vi "nanocal -- nuclear schottky fit V3.vi"() -> ()   [LabVIEW 2020] (continued)
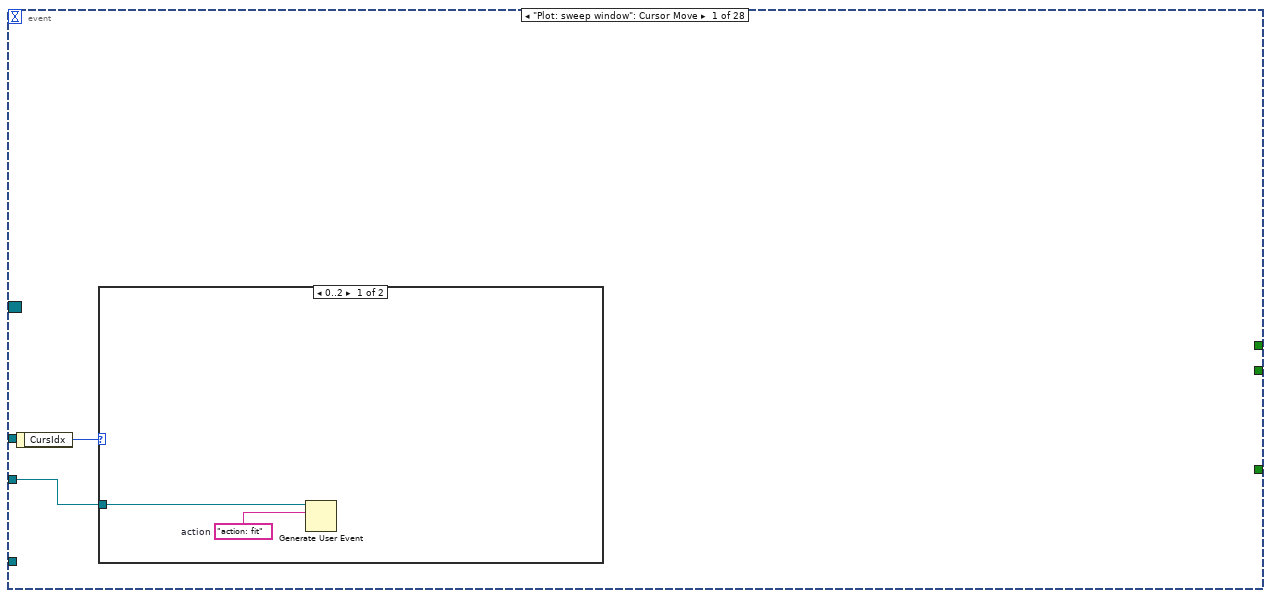
[diagram p2: hidden frame]
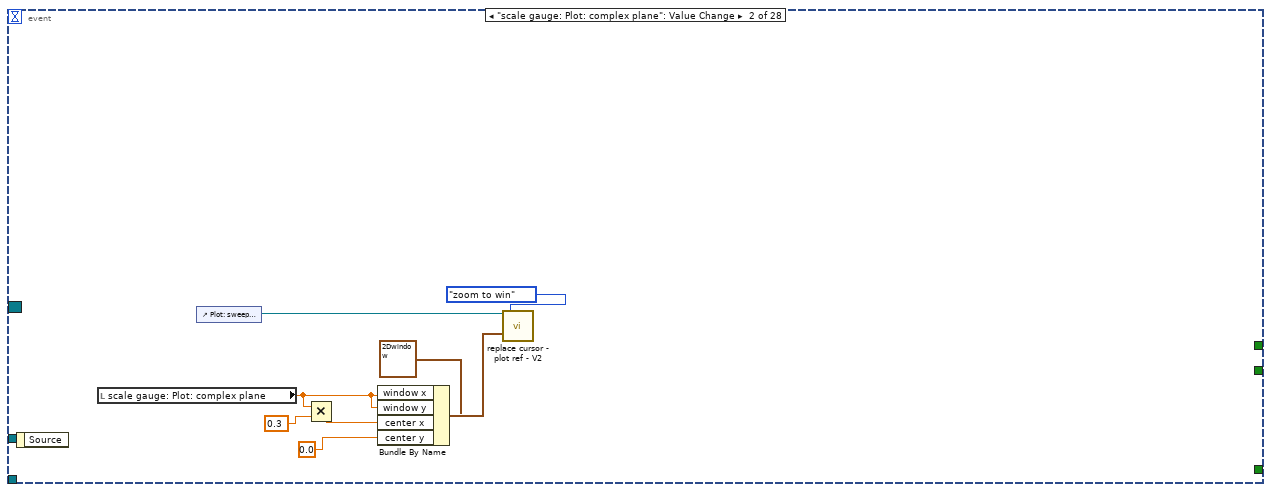
[diagram p4: hidden frame]
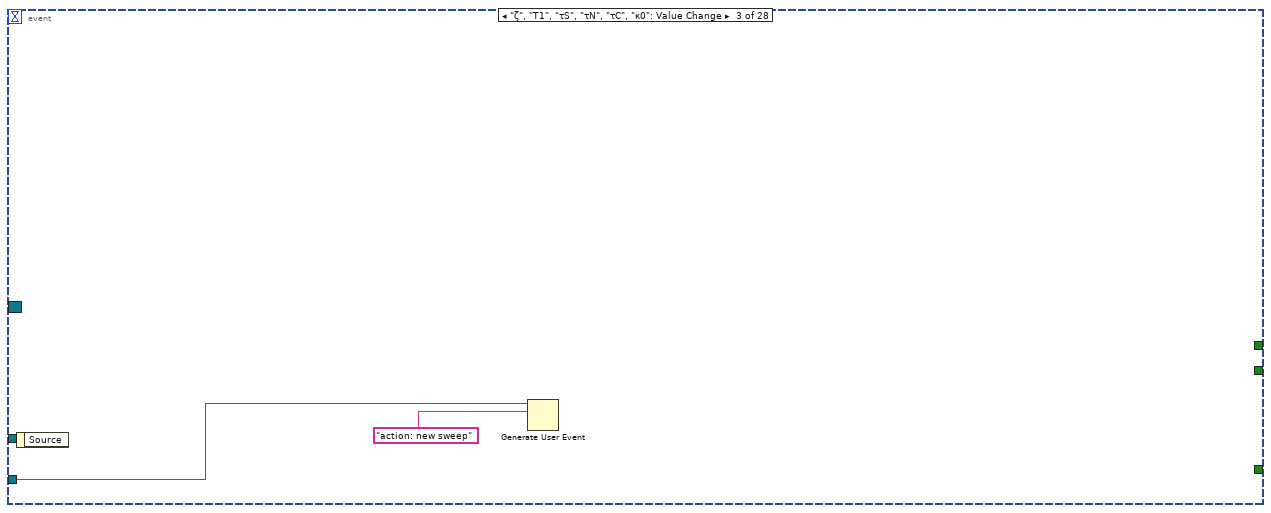
[diagram p5: hidden frame]
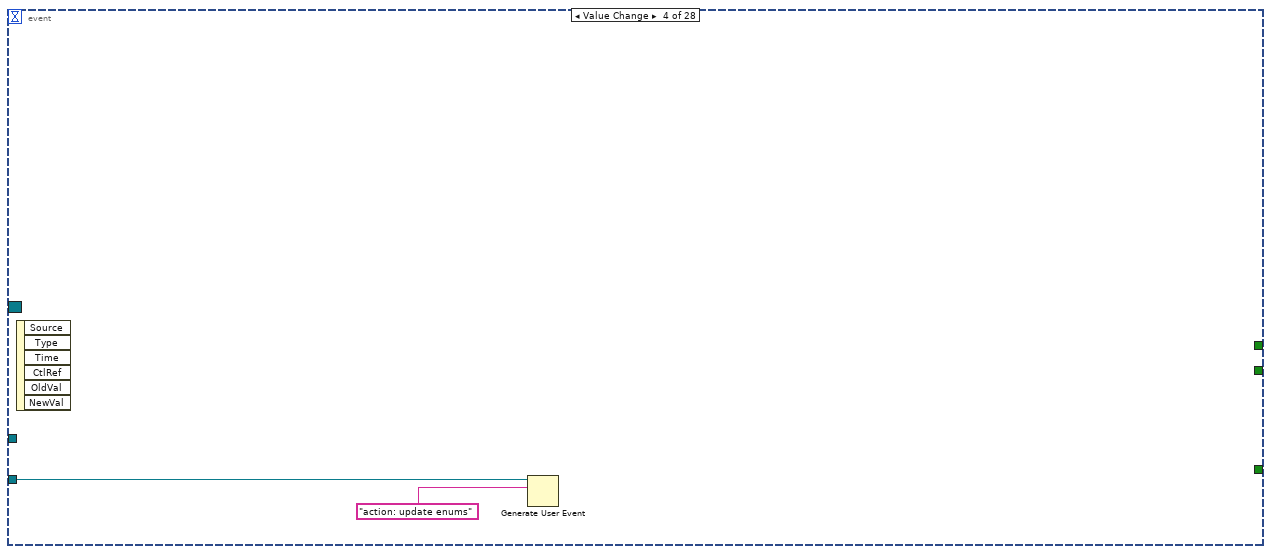
[diagram p6: hidden frame]
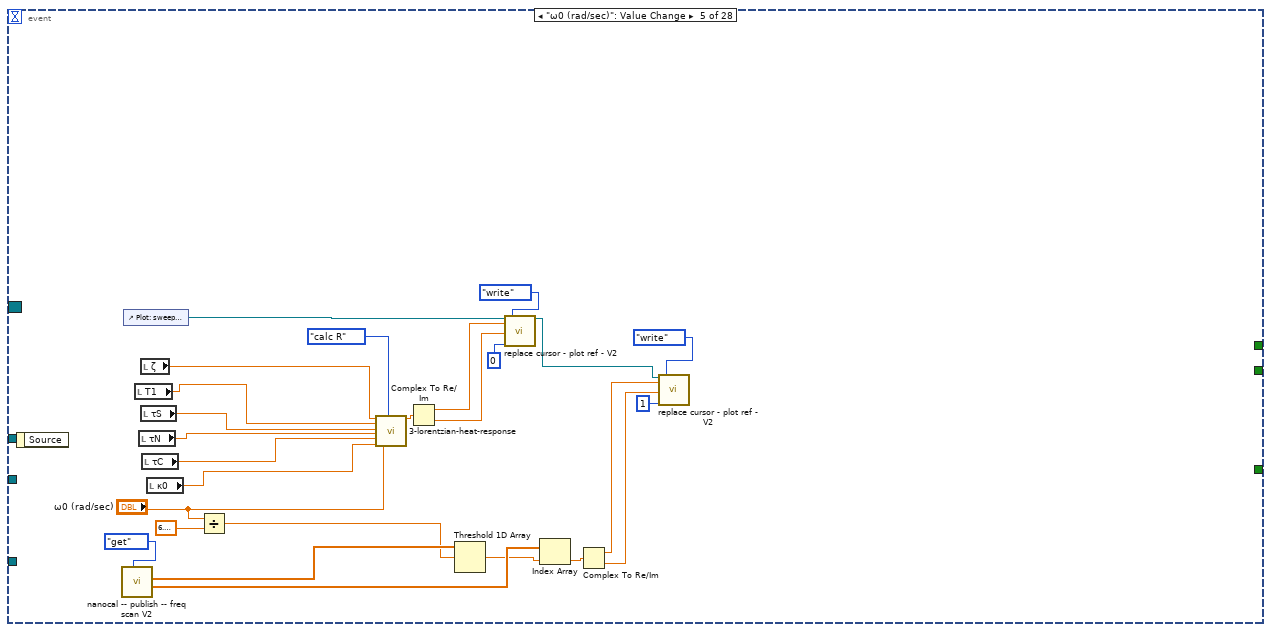
[diagram p7: hidden frame]
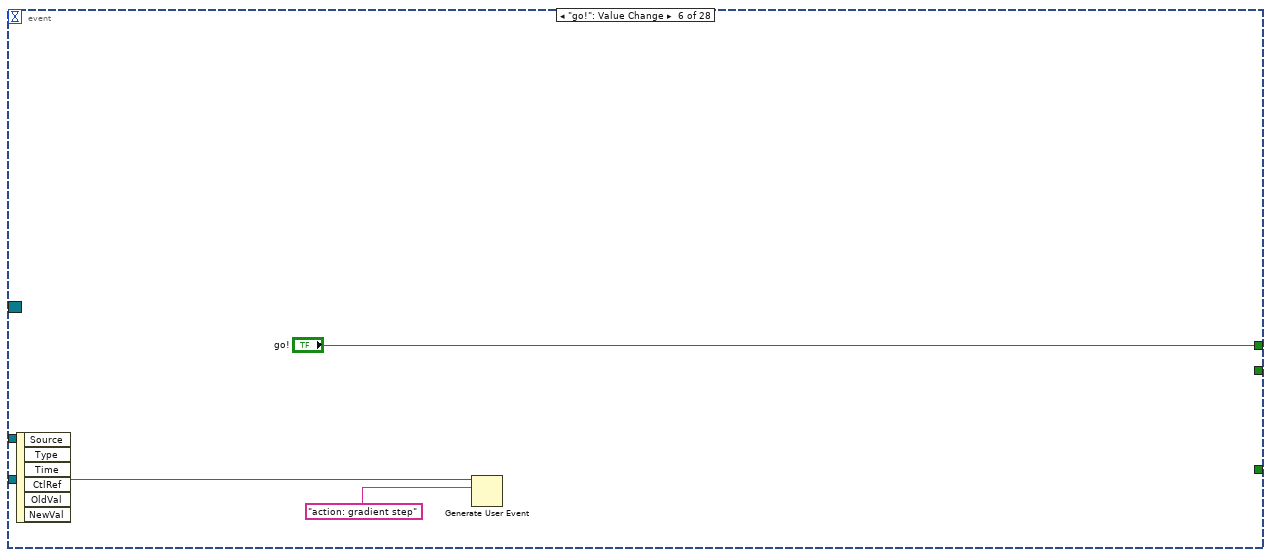
[diagram p8: hidden frame]
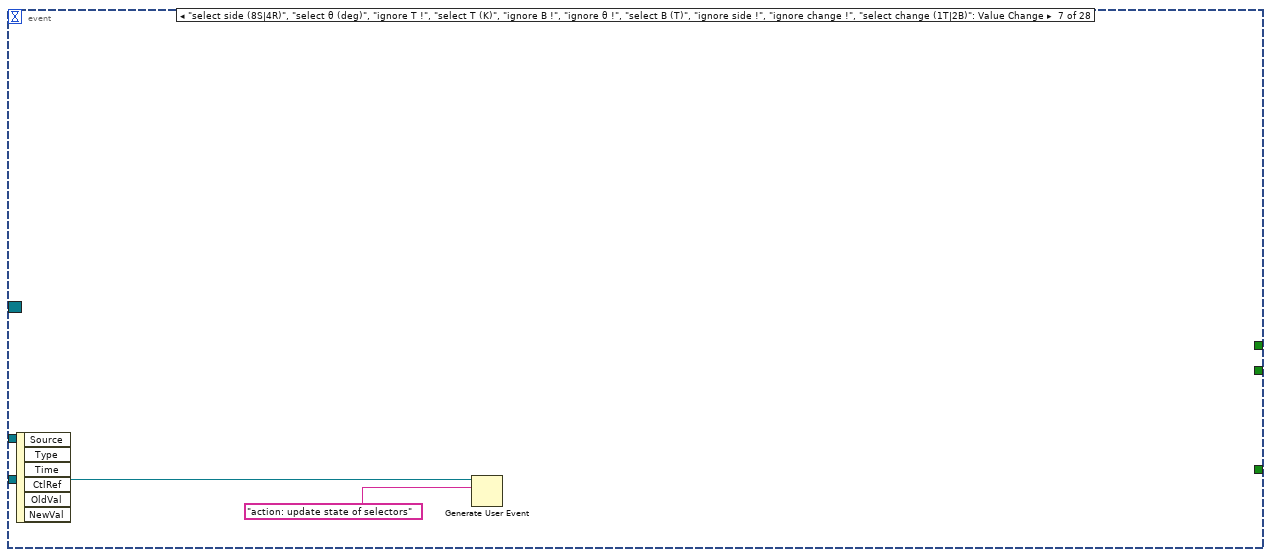
[diagram p9: hidden frame]
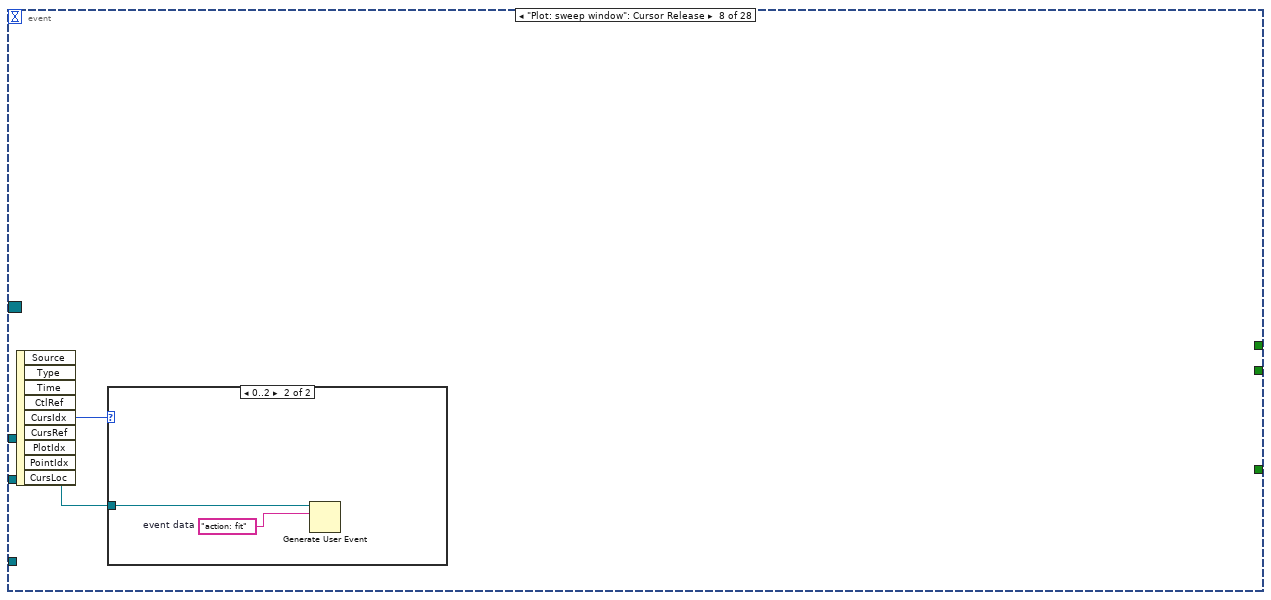
[diagram p10: hidden frame]
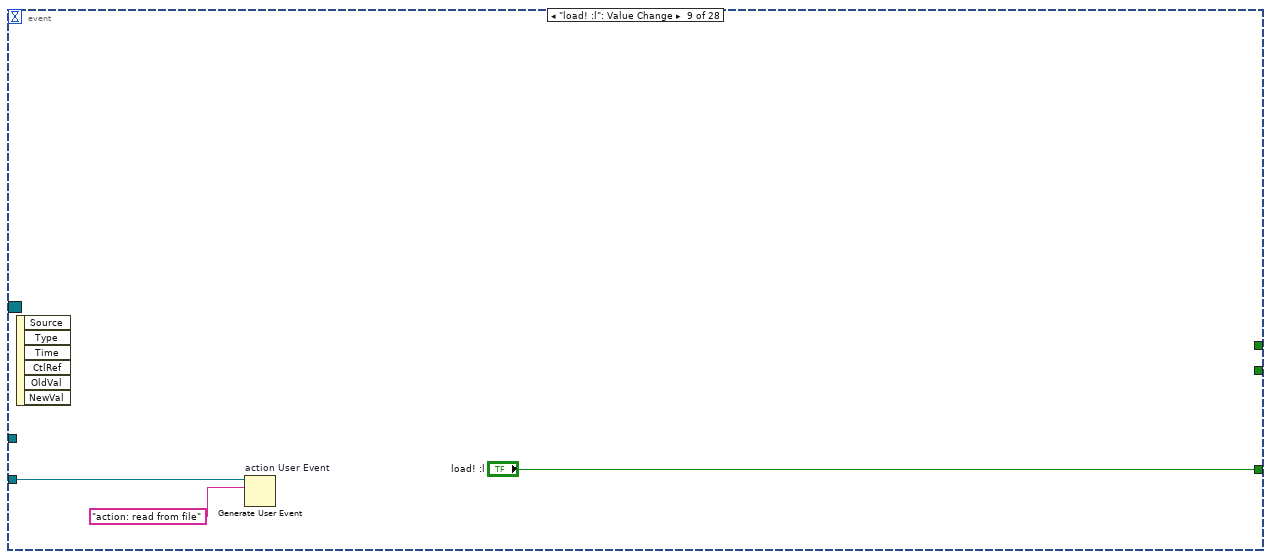
[diagram p12: hidden frame]
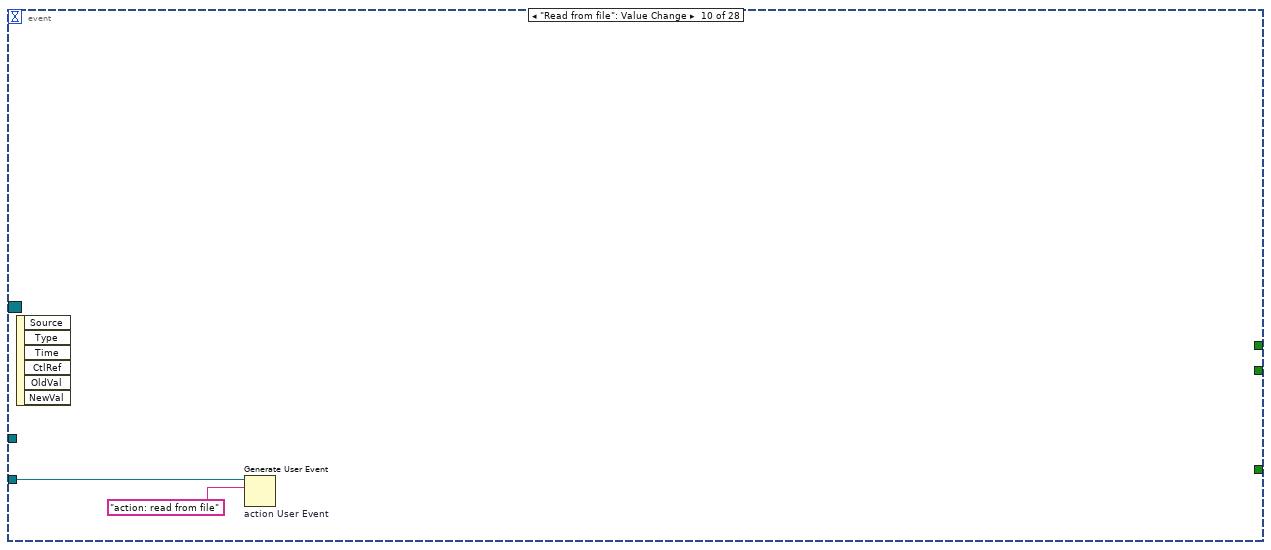
[diagram p13: hidden frame]
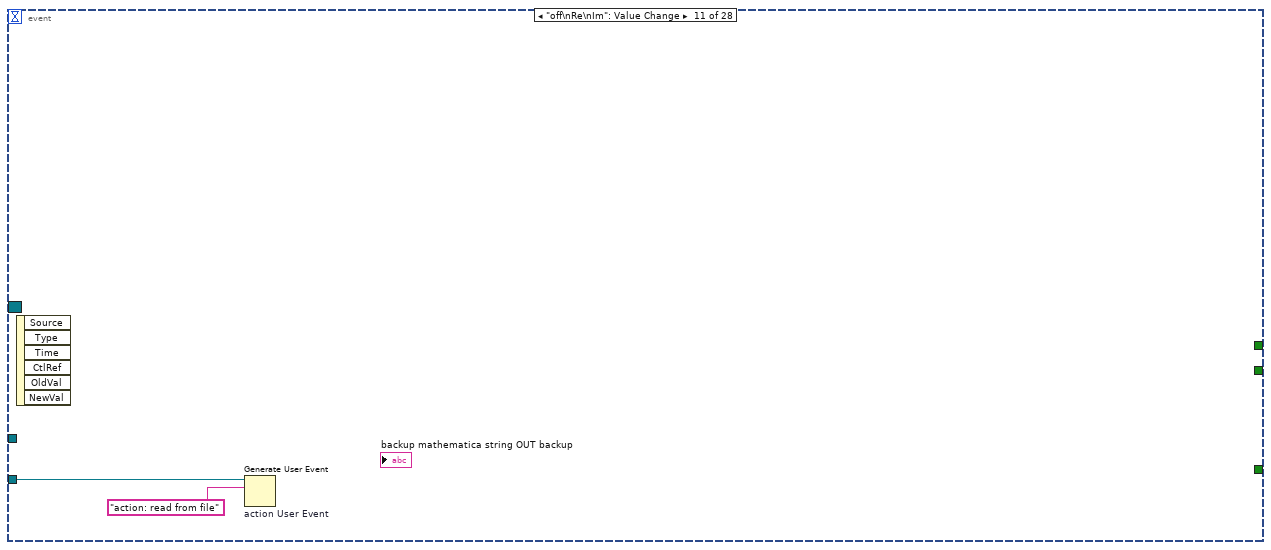
[diagram p14: hidden frame]
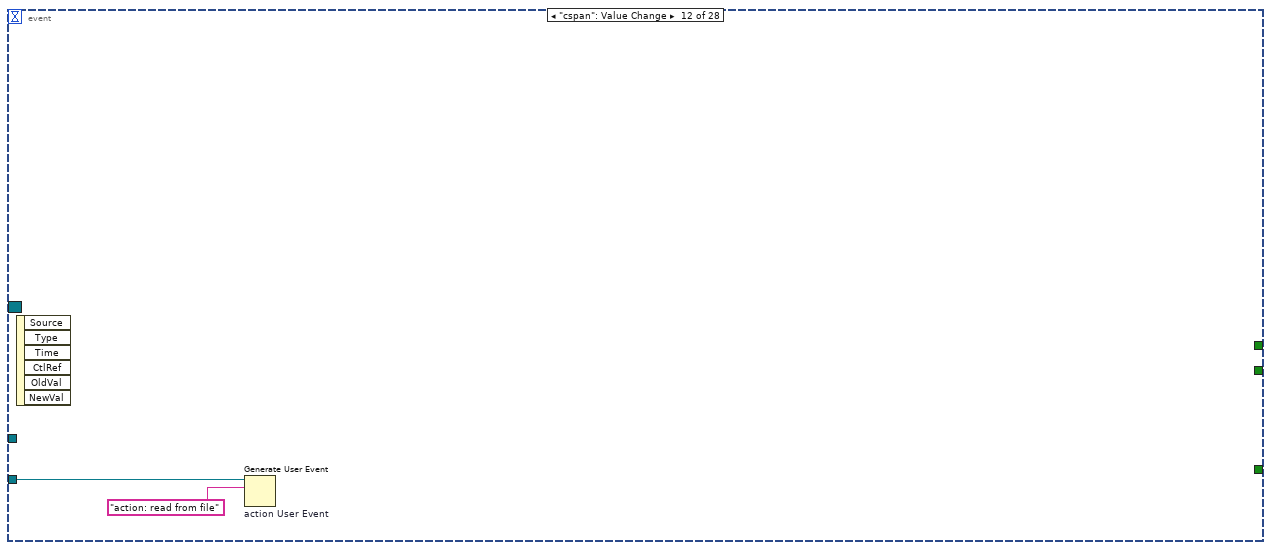
[diagram p15: hidden frame]
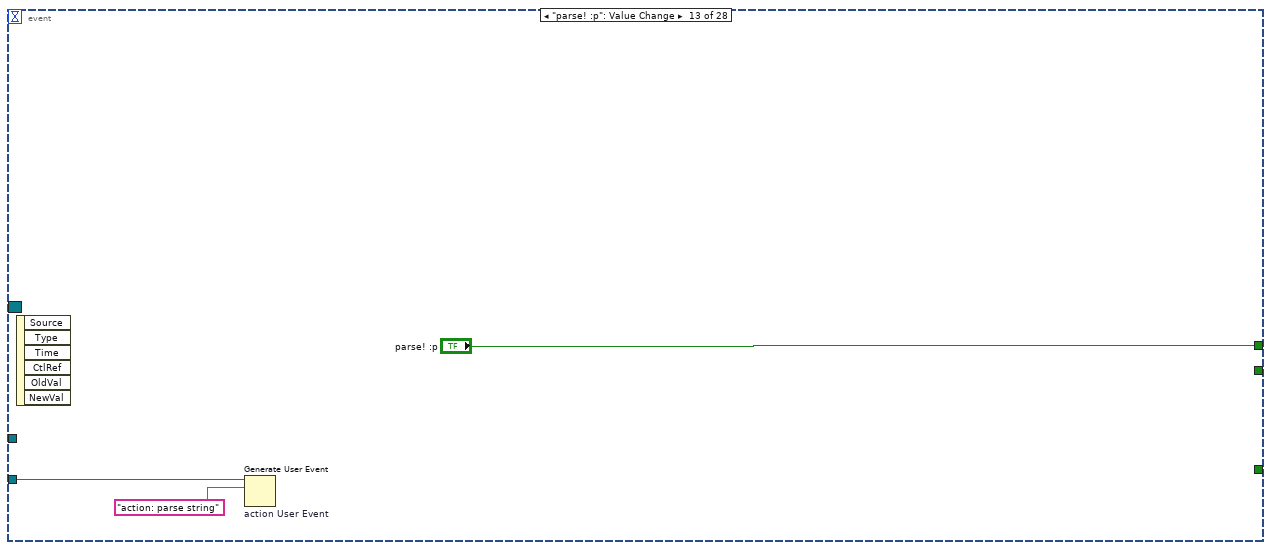
[diagram p16: hidden frame]
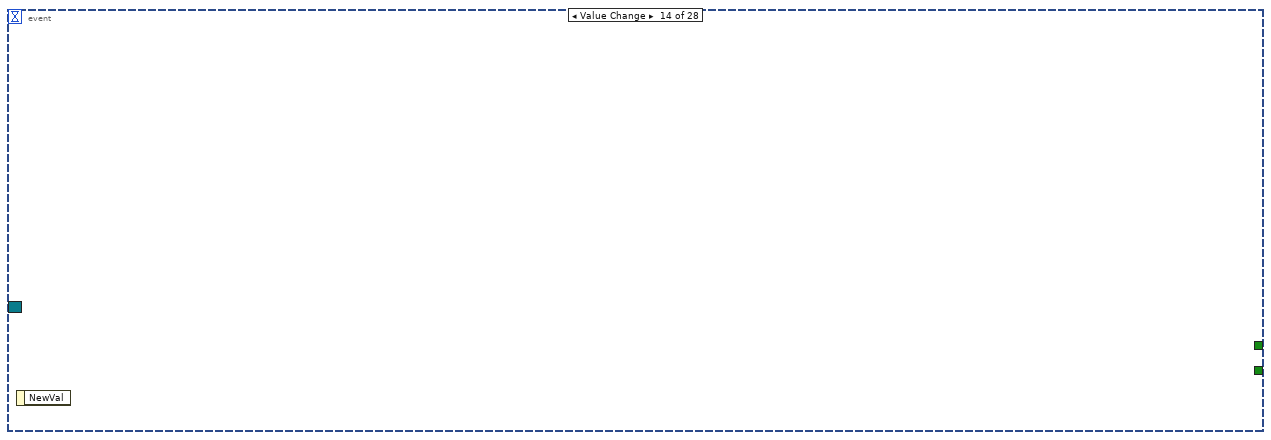
[diagram p17: hidden frame]
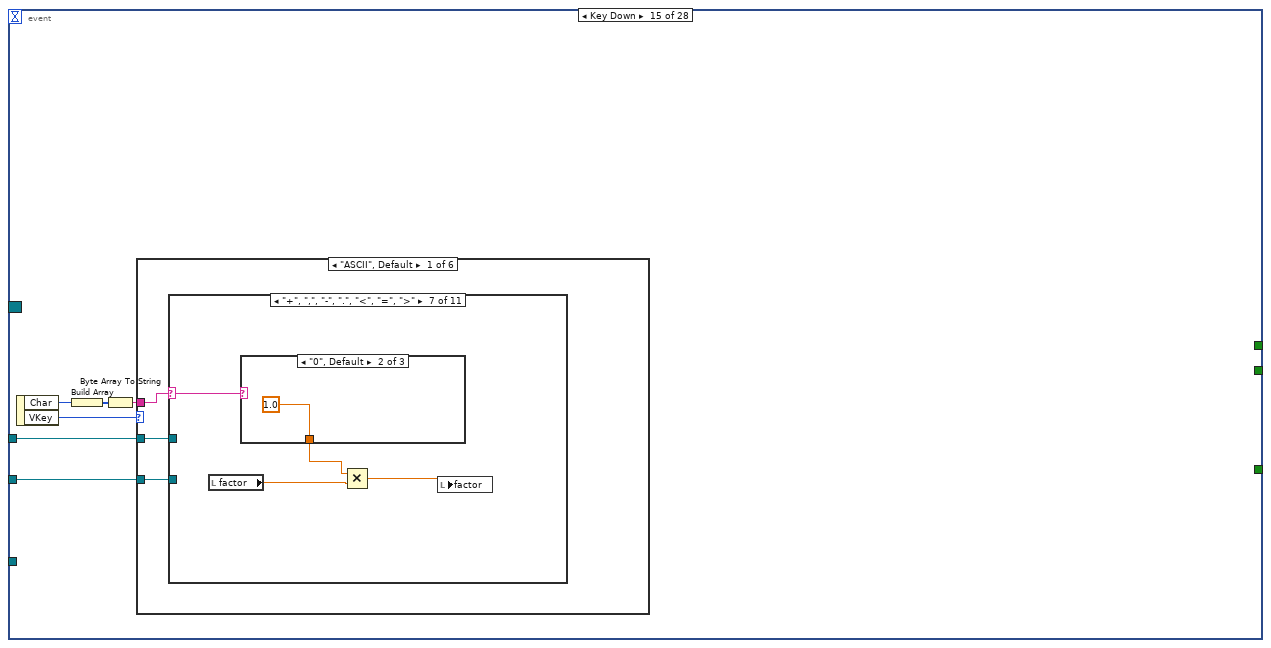
[diagram p18: hidden frame]
      event "ω0 (rad/sec)": Value Change {
        n583 = event-data() -> ()  [unwired: 1 in, 1 out]
        n584 = call "nanocal -- publish -- freq scan V2.vi"("publisher action"=publisher_action."get") -> ("z out (V)"=w1143:cdb[], "ω out (Hz)"=w1138:dbl[])  [unwired: 8 in, 1 out]
        n585 = control-ref of="Plot: sweep window"() -> (w1125:refnum<vi>)
        n586 = local read "T1"() -> (w1127:dbl)
        n587 = local read "τN"() -> (w1129:dbl)
        n588 = local read "ζ"() -> (w1126:dbl)
        n589 = local read "τS"() -> (w1128:dbl)
        n590 = local read "τC"() -> (w1130:dbl)
        n591 = local read "κ0"() -> (w1131:dbl)
        n592 = Divide(x="ω0 (rad/sec)", y=6.283185307179586) -> (x/y=w1136:dbl)
        n593 = call "3-lorentzian-heat-response.vi"("zeta"=w1126, "T1"=w1127, "tauS"=w1128, "tauN"=w1129, "tauC"=w1130, "kappa0"=w1131, "omega (rad/sec)"="ω0 (rad/sec)", "action"=3-lorentzian-heat-response_action."calc R") -> ("Romega"=w1134:cdb)  [unwired: 7 in, 4 out]
        n594 = Complex To Re/Im(x + iy=w1134) -> (x=w1132:dbl, y=w1133:dbl)
        n595 = Threshold 1D Array(2:w1136, 3:w1138) -> (0:w1137:dbl)  [unwired: 1 in]
        n596 = call "replace cursor - plot ref - V2.vi"("Plot ref in"=w1125, "new X"=w1132, "new  Y"=w1133, "cursor index"=0, "cursor action"=cursor_action."write") -> ("Plot ref out"=w1139:refnum<vi>)  [unwired: 11 in, 3 out]
        n597 = Index Array(array=w1143, index=w1137) -> (element=w1140:cdb)
        n598 = Complex To Re/Im(x + iy=w1140) -> (x=w1141:dbl, y=w1142:dbl)
        n599 = call "replace cursor - plot ref - V2.vi"("Plot ref in"=w1139, "new X"=w1141, "new  Y"=w1142, "cursor index"=1, "cursor action"=cursor_action."write") -> ()  [unwired: 11 in, 4 out]
      }
      event "go!": Value Change {
        n600 = event-data() -> ()  [unwired: 1 in, 6 out]
        n601 = Generate User Event(user event=w1145, event data cluster="action: gradient step" ("event data")) -> ()  [unwired: 2 in, 2 out]
      }
      event "select side (8S|4R)", "select θ (deg)", "ignore T !", "select T (K)", "ignore B !", "ignore θ !", "select B (T)", "ignore side !", "ignore change !", "select change (1T|2B)": Value Change {
        n602 = event-data() -> ()  [unwired: 1 in, 6 out]
        n603 = Generate User Event(user event=w1147, event data cluster="action: update state of selectors" ("event data")) -> ()  [unwired: 2 in, 2 out]
      }
      event "Plot: sweep window": Cursor Release {
        n604 = event-data() -> ("CursIdx"=w1149:i32)  [unwired: 1 in, 8 out]
        n605 = case shown="0..2" w1149 {
          tunnel: w1150 -> [_ w1151]
          frame 3, Default {
          }
          frame 0..2 {
            w1152 = "action: fit"  # event data
            n606 = Generate User Event(user event=w1151, event data cluster=w1152) -> ()  [unwired: 2 in, 2 out]
          }
        }
      }
      event "load! :l": Value Change {
        n607 = event-data() -> ()  [unwired: 1 in, 6 out]
        n608 = Generate User Event "action User Event"(user event=w1155, event data cluster="action: read from file" ("event data")) -> ()  [unwired: 2 in, 2 out]
      }
      event "Read from file": Value Change {
        n609 = event-data() -> ()  [unwired: 1 in, 6 out]
        n610 = Generate User Event "action User Event"(user event=w1156, event data cluster="action: read from file" ("event data")) -> ()  [unwired: 2 in, 2 out]
      }
      event "off\nRe\nIm": Value Change {
        n611 = event-data() -> ()  [unwired: 1 in, 6 out]
        n612 = Generate User Event "action User Event"(user event=w1158, event data cluster="action: read from file" ("event data")) -> ()  [unwired: 2 in, 2 out]
      }
      event "cspan": Value Change {
        n613 = event-data() -> ()  [unwired: 1 in, 6 out]
        n614 = Generate User Event "action User Event"(user event=w1160, event data cluster="action: read from file" ("event data")) -> ()  [unwired: 2 in, 2 out]
      }
      event "parse! :p": Value Change {
        n615 = event-data() -> ()  [unwired: 1 in, 6 out]
        n616 = Generate User Event "action User Event"(user event=w1163, event data cluster="action: parse string" ("event data")) -> ()  [unwired: 2 in, 2 out]
      }
      event Value Change {
        n617 = event-data() -> ()  [unwired: 1 in, 1 out]
      }
      event Key Down {
        n618 = event-data() -> ("Char"=w1167:i16, "VKey"=w1170:T28)  [unwired: 1 in]
        n619 = Build Array(w1167) -> (w1168:i16[])
        n620 = Byte Array To String(unsigned byte array=w1168) -> (string=w1166:string)
        n621 = case shown="\"ASCII\", Default" w1170 {
          selector: w1170 -> [_ _ _ _ _ w1202]
          tunnel: w1169 -> [w1173 _ _ w1198 _ _]
          tunnel: w1166 -> [w1172 _ _ _ _ _]
          tunnel: w1165 -> [w1171 _ _ _ _ w1201]
          frame "ASCII", Default {
            n622 = case shown="\"+\", \",\", \"-\", \".\", \"<\", \"=\", \">\"" w1172 {
              selector: w1172 -> [_ _ _ _ _ _ w1185 _ _ _ _]
              tunnel: w1173 -> [_ _ w1174 w1176 w1179 _ _ _ w1192 w1194 w1196]
              tunnel: w1171 -> [_ _ _ _ _ w1183 _ _ _ _ _]
              frame "0", Default {
              }
              frame "a" {
              }
              frame "s" {
                n623 = Generate User Event(user event=w1174, event data cluster="action: save freq scan" ("event data")) -> ()  [unwired: 2 in, 2 out]
              }
              frame "l" {
                n624 = Generate User Event(user event=w1176, event data cluster="action: read from file" ("event data")) -> ()  [unwired: 2 in, 2 out]
              }
              frame " " {
                n625 = Generate User Event(user event=w1179, event data cluster="action: gradient step" ("event data")) -> ()  [unwired: 2 in, 2 out]
              }
              frame "?" {
                # "?"
                n626 = call "replace cursor - plot ref - V2.vi"("Plot ref in"=w1183, "cursor action"=cursor_action."zoom to win") -> ("Plot ref out"=w1182:refnum<vi>)  [unwired: 14 in, 3 out]
                n627 = call "replace cursor - plot ref - V2.vi"("Plot ref in"=w1182, "cursor action"=cursor_action."smart zoom out&aspect") -> ()  [unwired: 14 in, 4 out]
              }
              frame "+", ",", "-", ".", "<", "=", ">" {
                n628 = local read "factor"() -> (w1187:dbl)
                n629 = case shown="\"0\", Default" w1185 {
                  tunnel: [0.7 1.0 1.5] -> w1184
                  frame ",", "-", "<" {
                  }
                  frame "0", Default {
                  }
                  frame "+", ".", "=", ">" {
                  }
                }
                n630 = Multiply(x=w1184, y=w1187) -> (x*y=w1186:dbl)
                n631 = local write "factor"(w1186) -> ()
              }
              frame "b" {
                n632 = local read "String"() -> (w1191:string)
                n633 = local write "backup string :b"(w1191) -> ()
              }
              frame "u" {
                n634 = Generate User Event(user event=w1192, event data cluster="ignoreaction: uco" ("event data")) -> ()  [unwired: 2 in, 2 out]
              }
              frame "p" {
                n635 = Generate User Event "action User Event"(user event=w1194, event data cluster="action: parse string" ("event data")) -> ()  [unwired: 2 in, 2 out]
              }
              frame "m" {
                n636 = Generate User Event "action User Event"(user event=w1196, event data cluster="action: copy from math" ("event data")) -> ()  [unwired: 2 in, 2 out]
              }
            }
          }
          frame "Escape" {
          }
          frame "PageUp" {
          }
          frame "Enter" {
            n637 = Generate User Event "action User Event"(user event=w1198, event data cluster="action: replot colors" ("event data")) -> ()  [unwired: 2 in, 2 out]
            n638 = Generate User Event "action User Event"(user event=w1198, event data cluster="action: new sweep" ("event data")) -> ()  [unwired: 2 in, 2 out]
          }
          frame "PageDown" {
          }
          frame "Up".."Right" {
            n639 = case shown="\"Down\"" w1202 {
              tunnel: [cursor_action."zoom in 20%" ("cursor action") cursor_action."zoom out 20%" ("cursor action") cursor_action."zoom out 20%" ("cursor action") cursor_action."zoom in 20%" ("cursor action")] -> w1203
              frame "Up", Default {
              }
              frame "Down" {
              }
              frame "Left" {
              }
              frame "Right" {
              }
            }
            n640 = call "replace cursor - plot ref - V2.vi"("Plot ref in"=w1201, "cursor action"=w1203) -> ()  [unwired: 14 in, 4 out]
          }
        }
      }
      event "Plot:  colors": Cursor Move {
        n641 = event-data() -> ("CursIdx"=w1211:i32)  [unwired: 1 in]
        n642 = local read "T1"() -> (w1227:dbl)
        n643 = local read "τS"() -> (w1228:dbl)
        n644 = local read "τN"() -> (w1229:dbl)
        n645 = local read "τC"() -> (w1230:dbl)
        n646 = local read "κ0"() -> (w1231:dbl)
        n647 = local read "ζ"() -> (w1226:dbl)
        n648 = call "replace cursor - plot ref - V2.vi"("Plot ref in"=w1232, "cursor index"=w1211, "cursor action"=cursor_action."read") -> ("read Y"=w1210:dbl)  [unwired: 13 in, 3 out]
        n649 = Build Array(w1226, w1227, w1228, w1229, w1230, w1231) -> (w1213:dbl[])
        n650 = Replace Array Subset(array=w1213, new element=w1210, index=w1211) -> (w1212:dbl[])
        n651 = Generate User Event(user event=w1209, event data cluster="action: replot circles" ("event data")) -> ()  [unwired: 2 in, 2 out]
        n652 = Index Array(array=w1212, index #1=0 ("index"), index #2=1 ("index"), index #3=2 ("index"), index #4=3 ("index"), index #5=4 ("index"), index #6=5 ("index")) -> (element #1=w1219:dbl, element #2=w1218:dbl, element #3=w1217:dbl, element #4=w1216:dbl, element #5=w1215:dbl, element #6=w1214:dbl)
        n653 = local write "τN"(w1216) -> ()
        n654 = local write "τC"(w1215) -> ()
        n655 = local write "τS"(w1217) -> ()
        n656 = local write "κ0"(w1214) -> ()
        n657 = local write "T1"(w1218) -> ()
        n658 = local write "ζ"(w1219) -> ()
      }
      event "pause!": Value Change {
        n659 = event-data() -> ()  [unwired: 1 in, 6 out]
        n660 = local write "newton pause"(TRUE ("newton pause")) -> ()
      }
      event "uco! :u": Value Change {
        n661 = event-data() -> ()  [unwired: 1 in, 1 out]
        n662 = Generate User Event(user event=w1237, event data cluster="ignoreaction: uco" ("event data")) -> ()  [unwired: 2 in, 2 out]
      }
      event "Read  τ's  from  Math !": Value Change {
        n663 = event-data() -> ()  [unwired: 1 in, 1 out]
        n664 = Generate User Event(user event=w1240, event data cluster="action: copy from math" ("event data")) -> ()  [unwired: 2 in, 2 out]
      }
      event "Write τ's to  Math!": Value Change {
        n665 = event-data() -> ()  [unwired: 1 in, 1 out]
        n666 = Generate User Event(user event=w1243, event data cluster="action: copy to math" ("event data")) -> ()  [unwired: 2 in, 2 out]
      }
      event "Math --> string OUT!": Value Change {
        n667 = event-data() -> ()  [unwired: 1 in, 1 out]
        n668 = Generate User Event(user event=w1246, event data cluster="action: write mathematica string" ("event data")) -> ()  [unwired: 2 in, 2 out]
      }
      event "generate empty string from filelist": Value Change {
        n669 = event-data() -> ()  [unwired: 1 in, 1 out]
        n670 = Generate User Event(user event=w1249, event data cluster="action: empty string from filelist" ("event data")) -> ()  [unwired: 2 in, 2 out]
      }
      event "string IN  --> Math!": Value Change {
        n671 = event-data() -> ()  [unwired: 1 in, 1 out]
        n672 = Generate User Event(user event=w1252, event data cluster="action: read mathematica string" ("event data")) -> ()  [unwired: 2 in, 2 out]
      }
      event "filenames": Value Change {
        n673 = event-data() -> ()  [unwired: 1 in, 6 out]
        n674 = local read "filesnames lookup"() -> (w1260:map{i32, i32})
        n675 = local read "filenames"() -> (w1258:map{i32, string})
        n676 = local read "filenames"() -> (w1259:u16)
        n677 = local read "folder"() -> (w1261:path)
        n678 = Look In Map(map=w1260, key=w1259) -> (value=w1257:i32)  [unwired: 1 in, 1 out]
        n679 = Look In Map(map=w1258, key=w1257) -> (value=w1256:string)  [unwired: 1 in, 1 out]
        n680 = Build Path(base path=w1261, name or relative path=w1256) -> (appended path=w1254:path)
        n681 = for {
          N: 1 -> [_]
          tunnel: w1262 -> [w1264]
          tunnel: w1254 -> [w1263]
          n682 = local write "Read from file"(w1263) -> ()
          n683 = Generate User Event(user event=w1264, event data cluster="action: read from file" ("event data")) -> ()  [unwired: 2 in, 2 out]
        }
      }
      event "constrained filenames": Value Change {
        n684 = event-data() -> ()  [unwired: 1 in, 6 out]
        n685 = local read "constrained filename lookup"() -> (w1272:map{i32, i32})
        n686 = local read "constrained filenames"() -> (w1271:u16)
        n687 = local read "filenames"() -> (w1270:map{i32, string})
        n688 = local read "folder"() -> (w1273:path)
        n689 = Look In Map(map=w1272, key=w1271) -> (value=w1269:i32)  [unwired: 1 in, 1 out]
        n690 = Look In Map(map=w1270, key=w1269) -> (value=w1268:string)  [unwired: 1 in, 1 out]
        n691 = Build Path(base path=w1273, name or relative path=w1268) -> (appended path=w1266:path)
        n692 = for {
          N: 1 -> [_]
          tunnel: w1274 -> [w1276]
          tunnel: w1266 -> [w1275]
          n693 = local write "Read from file"(w1275) -> ()
          n694 = Generate User Event(user event=w1276, event data cluster="action: read from file" ("event data")) -> ()  [unwired: 2 in, 2 out]
        }
      }
      event User Event {
        n695 = event-data() -> ("interface"=w1279:string)  [unwired: 1 in, 4 out]
        n696 = case shown="\"interface: update color cursors\"" w1279 {
          tunnel: [_ _ TRUE] -> w1278
          frame "void", Default {
          }
          frame "interface: update color cursors" {
            w1283 = T1[] [enum."T (K)", enum."B (T)", enum."θ (deg)"] items=["ζ", "τ1", "τS", "τN", "τC", "κ0", "m1", "m2", "m3", "T (K)", "B (T)", "θ (deg)", "side (S|R)", "change (B|T)"]
            w1280 = T1[] [enum."ζ", enum."τ1", enum."τS", enum."τN", enum."τC", enum."κ0", enum."m1", enum."m2", enum."m3"] items=["ζ", "τ1", "τS", "τN", "τC", "κ0", "m1", "m2", "m3", "T (K)", "B (T)", "θ (deg)", "side (S|R)", "change (B|T)"]
            n697 = local read "T1"() -> (w1291:dbl)
            n698 = local read "τS"() -> (w1292:dbl)
            n699 = local read "τN"() -> (w1293:dbl)
            n700 = local read "τC"() -> (w1294:dbl)
            n701 = local read "κ0"() -> (w1295:dbl)
            n702 = local read "ζ"() -> (w1290:dbl)
            n703 = Build Array(w1290, w1291, w1292, w1293, w1294, w1295) -> (w1297:dbl[])
            n704 = for {
              shift-right: [w1313] -> w1298
              shift-left: map{T1, dbl} {} ("Map IN") -> [w1314]
              tunnel: w1280 -> [w1311] mode=indexing
              tunnel: w1297 -> [w1312] mode=indexing
              tunnel: [w1311] -> w1306 mode=indexing
              n705 = Insert Into Map(map in=w1314, key=w1311, value=w1312) -> (map out=w1313:map{T1, dbl})  [unwired: 2 out]
            }
            n706 = call "3-lorentzian-heat-response -- V4.vi"("action"=3-lorentzian-heat-response_action."calc m1m2m3", "Map IN"=w1298) -> ("Map OUT"=w1302:map{T1, dbl})  [unwired: 7 in, 2 out]
            n707 = local read "θ (deg)"() -> (w1301:dbl)
            n708 = local read "B (T)"() -> (w1300:dbl)
            n709 = local read "T (K)"() -> (w1299:dbl)
            n710 = local read "cursor x selector"() -> (w1286:map{T1, dbl})
            n711 = Build Array(w1299, w1300, w1301) -> (w1303:dbl[])
            n712 = local read "X selector"() -> (w1287:T1)
            n713 = local read "cursor index map"() -> (w1296:map{T1, i32})
            n714 = local read "T (K)"() -> (w1288:dbl)
            n715 = for {
              shift-right: [w1309] -> w1304
              shift-left: w1302 -> [w1310]
              tunnel: w1283 -> [w1308] mode=indexing
              tunnel: w1303 -> [w1307] mode=indexing
              n716 = Insert Into Map(map in=w1310, key=w1308, value=w1307) -> (map out=w1309:map{T1, dbl})  [unwired: 2 out]
            }
            n717 = control-ref of="Plot:  colors"() -> (w1285:refnum<vi>)
            n718 = Look In Map(map=w1286, key=w1287, default value=w1288) -> (value=w1289:dbl)  [unwired: 1 out]
            n719 = for {
              tunnel: w1289 -> [w1322]
              tunnel: w1285 -> [w1321]
              tunnel: w1306 -> [w1317] mode=indexing
              tunnel: w1296 -> [w1319]
              shift-right: [w1316] -> _
              shift-left: w1302 -> [w1316]
              n720 = Look In Map(map=w1316, key=w1317) -> (value=w1315:dbl)  [unwired: 1 in, 1 out]
              n721 = Look In Map(map=w1319, key=w1317) -> (value=w1318:i32)  [unwired: 1 in, 1 out]
              n722 = call "replace cursor - plot ref - V2.vi"("Plot ref in"=w1321, "new X"=w1322, "new  Y"=w1315, "cursor index"=w1318, "cursor action"=cursor_action."write") -> ()  [unwired: 11 in, 4 out]
            }
            n723 = call "string parse mathematica assosiated array.vi"("derivative"=mathematica_string_map_action."create string", "Map IN"=w1304) -> ("String OUT"=w1305:string)  [unwired: 8 in, 1 out]
            n724 = local write "String"(w1305) -> ()
          }
          frame "interface: exit" {
          }
        }
      }
      event "plot landscape!", "range one", "range two": Value Change {
        n725 = event-data() -> ()  [unwired: 1 in, 6 out]
        n726 = Generate User Event(user event=w1324, event data cluster="action: plot landscape" ("event data")) -> ()  [unwired: 2 in, 2 out]
      }
      event "colors": Value Change {
        n727 = event-data() -> ()  [unwired: 1 in, 6 out]
        n728 = Generate User Event(user event=w1327, event data cluster="action: reset colors" ("event data")) -> ()  [unwired: 2 in, 2 out]
      }
    }
  }
  "cursor x selector" <- w23
